vi "Test API Throws Error if Path to VI.vi"(8 "error in (no error)":errorcluster, 11 "API Test in":refnum<class "API Test.lvclass">) -> (0 "error out":errorcluster, 3 "API Test out":refnum<class "API Test.lvclass">)   [LabVIEW 2020, in "LUnit Tests.lvlib" / "API Test.lvclass"]
uses:
  API Test.lvclass
  source/Framework/Execution API/Execution API.lvclass
  <vilib>/Astemes/LUnit/Test Case.lvclass
  C:/Program Files (x86)/National Instruments/LabVIEW 2021/vi.lib/Astemes/LUnit/Test Case.lvclass
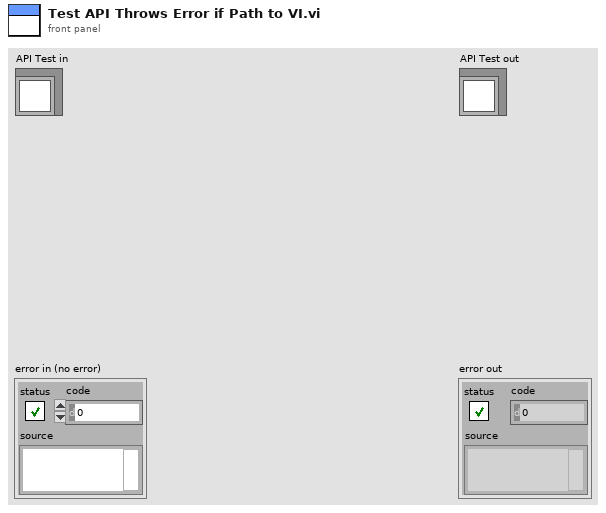
[diagram p1: front panel]
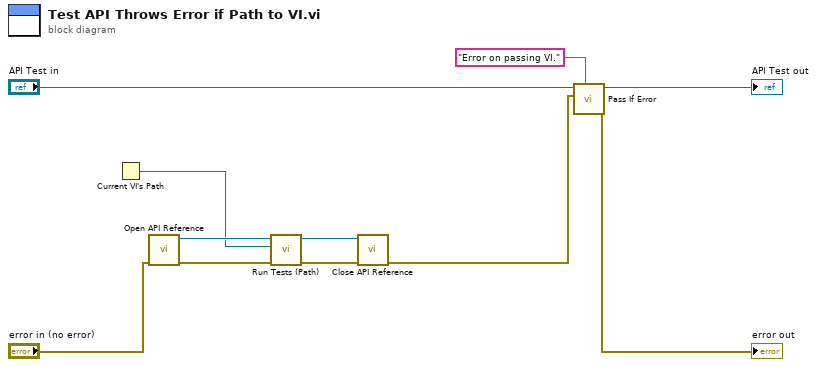
[diagram p0: block diagram]
diagram:
  n1 = Current VI's Path() -> (path=w1:path)
  n2 = call "Open API Reference.vi"("error in (no error)"="error in (no error)") -> ("error out"=w10:errorcluster, "Execution API out"=w11:refnum<class "Execution API.lvclass">)  [unwired: 9 in]
  n3 = call "Run Tests (Path).vi"("error in (no error)"=w10, "Project or Class Path"=w1, "Execution API In"=w11) -> ("error out"=w9:errorcluster, "Execution API Out"=w8:refnum<class "Execution API.lvclass">)  [unwired: 7 in]
  n4 = call "Close API Reference.vi"("error in (no error)"=w9, "Execution API in"=w8) -> ("error out"=w4:errorcluster)  [unwired: 9 in]
  n5 = call <vilib>:"Pass If Error.vi"("Description"="Error on passing VI.", "Assert error"=w4, "LUnit Test Case In"="API Test in") -> ("error out"=→"error out":errorcluster, "LUnit Test Case Out"=→"API Test out":refnum<class "API Test.lvclass">)  [unwired: 7 in]
